vi "AlliGator Compute Average Plot Phasor.vi"(8 "error in (no error)":errorcluster, 9 "Phasor Frequency":dbl[unit]=160000000.0 format="%#_4g", 10 "Mouse Click Coordinates":T2, 11 "XYGraph Ref":refnum<vi>) -> (0 "error out":errorcluster, 1 "Result String":string, 2 "Phasor SDV (g, s)":T1, 3 "Phasor (g, s)":T1)   [LabVIEW 2021, in "AlliGator Phasor Graph.lvlib"]
doc: "Computes average phasor of a single, selected or all phasor plots in the Phasor Graph."
uses:
  AlliGator Phasor Graph.lvlib
  <vilib>/Utility/miscctls.llb/LVPoint32TypeDef.ctl
  Phasor/Phasor (g, s).ctl
  Graphs/Get Plot at Mouse Click (XY Graph)/Get Plot at Mouse Click [AAC].vi
  <userlib>/_OpenG.lib/array/array.llb/Filter 1D Array with Scalar (I32)__ogtk.vi
  <userlib>/_OpenG.lib/array/array.llb/Filter 1D Array (DBL)__ogtk.vi
  Graphs/Graphs.lvlib
  Phasor/Phasor.lvlib
  <vilib>/Analysis/NI_AALBase.lvlib
  Arrays/Arrays.lvlib
  Strings/Strings.lvlib
  Graphs/XY Graph/XY Graph Add-Ons.lvlib
  Phasor Ratio/AlliGator Phasor Ratio.lvlib
  <userlib>/_OpenG.lib/array/array.llb/openg_array.lvlib
  Utilities/Utilities.lvlib
panel:
  # "see the AlliGator License on the block diagram (Ctrl+E or Window:Show Block Diagram)"
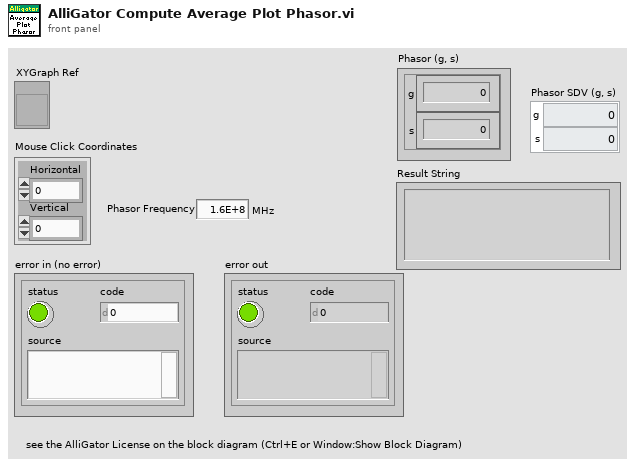
[diagram p1: front panel]
types:
  T1 = typedef "Phasor.lvlib/Phasor (g, s).ctl" = cluster{"g":dbl, "s":dbl}
  T2 = typedef "LVPoint32TypeDef.ctl" = cluster{"Horizontal":i32, "Vertical":i32}
  T3 = typedef "XY Graph Add-Ons.lvlib/XY Graph Refnum.ctl" = refnum<vi>
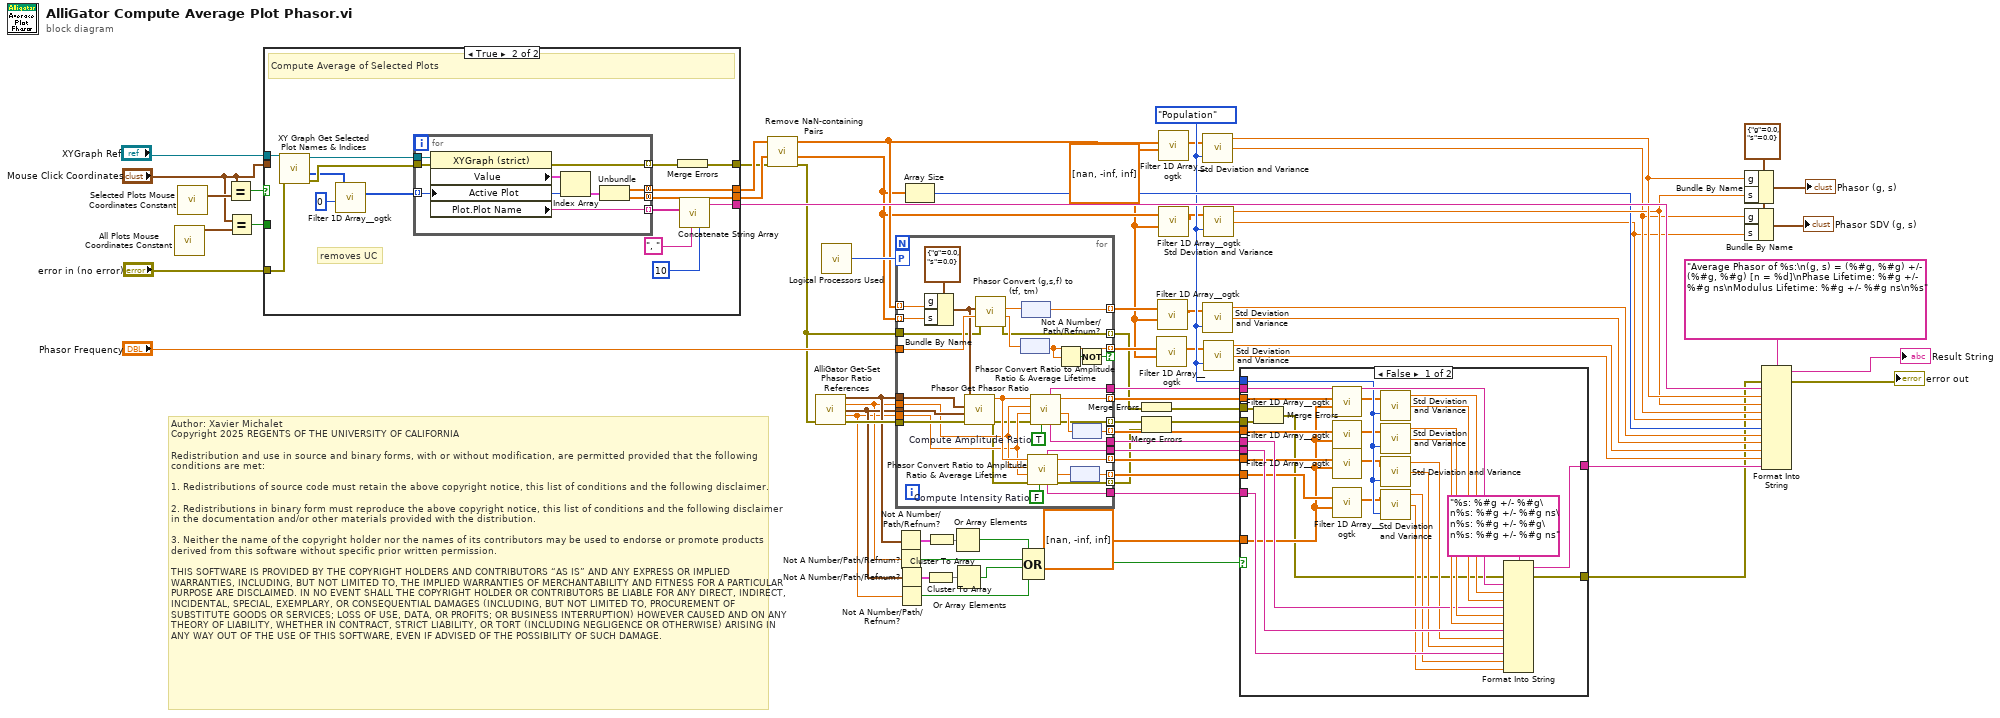
[diagram p0: block diagram]
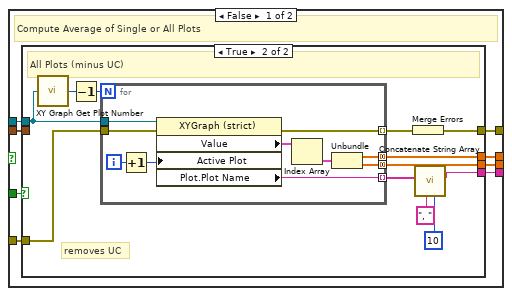
[diagram p3: hidden frame]
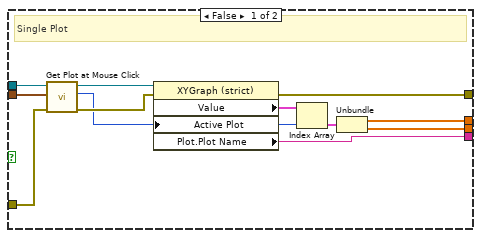
[diagram p4: hidden frame]
diagram:
  w9 = dbl[] [nan, -inf, inf] ("Element(s) to Remove")
  w29 = enum16{"Sample", "Population"}."Population" ("Weighting (Sample)")
  w50 = T1 {"g"=0.0, "s"=0.0} ("Phasor (g, s)")
  # "Author: Xavier Michalet\nCopyright 2025 REGENTS OF THE UNIVERSITY OF CALIFORNIA\n\nRedistribution and use in source and binary forms, with or without modification, are permitted provided that the following conditions are met:\n\n1. Redistributions of source code must retain the above copyright notice, this list of conditions and the following disclaimer.\n\n2. Redistributions in binary form must reproduce the above copyright notice, this list of conditions and the following disclaimer in the documentation and/or other materials provided with the distribution.\n\n3. Neither the name of the copyright holder nor the names of its contributors may be used to endorse or promote products derived from this software without specific prior written permission.\n\nTHIS SOFTWARE IS PROVIDED BY THE COPYRIGHT HOLDERS AND CONTRIBUTORS “AS IS” AND ANY EXPRESS OR IMPLIED WARRANTIES, INCLUDING, BUT NOT LIMITED TO, THE IMPLIED WARRANTIES OF MERCHANTABILITY AND FITNESS FOR A PARTICULAR PURPOSE ARE DISCLAIMED. IN NO EVENT SHALL THE COPYRIGHT HOLDER OR CONTRIBUTORS BE LIABLE FOR ANY DIRECT, INDIRECT, INCIDENTAL, SPECIAL, EXEMPLARY, OR CONSEQUENTIAL DAMAGES (INCLUDING, BUT NOT LIMITED TO, PROCUREMENT OF SUBSTITUTE GOODS OR SERVICES; LOSS OF USE, DATA, OR PROFITS; OR BUSINESS INTERRUPTION) HOWEVER CAUSED AND ON ANY THEORY OF LIABILITY, WHETHER IN CONTRACT, STRICT LIABILITY, OR TORT (INCLUDING NEGLIGENCE OR OTHERWISE) ARISING IN ANY WAY OUT OF THE USE OF THIS SOFTWARE, EVEN IF ADVISED OF THE POSSIBILITY OF SUCH DAMAGE."
  n1 = call "All Plots Mouse Coordinates Constant.vi"() -> ("Selected Plots Mouse Coordinates Equivalent"=w2:T2)
  n2 = call "Selected Plots Mouse Coordinates Constant.vi"() -> ("Selected Plots Mouse Coordinates Equivalent"=w54:T2)
  n3 = Equal?(x="Mouse Click Coordinates", y=w54) -> (x = y?=w53:bool)
  n4 = Equal?(x="Mouse Click Coordinates", y=w2) -> (x = y?=w1:bool)
  n5 = case shown="True" w53 {
    tunnel: "XYGraph Ref" -> [w77 w119]
    tunnel: "error in (no error)" -> [w76 w116]
    tunnel: [w75 w121] -> w66
    tunnel: [w74 w126] -> w62
    tunnel: [w73 w125] -> w61
    tunnel: [w72 w123] -> w60
    tunnel: "Mouse Click Coordinates" -> [w71 _]
    tunnel: w1 -> [w70 _]
    frame False {
      # "Compute Average of Single or All Plots"
      n6 = case shown="True" w70 {
        tunnel: w77 -> [w89 w93]
        tunnel: w76 -> [w88 w92]
        tunnel: [w82 w94] -> w75
        tunnel: [w81 w96] -> w74
        tunnel: [w80 w95] -> w73
        tunnel: [w79 w97] -> w72
        tunnel: w71 -> [w78 _]
        frame False {
          # "Single Plot"
          n7 = call-poly "Get Plot at Mouse Click.vi"("error in (no error)"=w88, "Mouse Click Coordinates"=w78, "XYGraph Ref"=w89) -> ("error out"=w86:errorcluster, "Plot at Coordinates"=w83:i32, "XYGraph Ref"=w87:T3)  [unwired: 2 in, 4 out]
          n8 = property class="XYGraph (strict)"(reference=w87, error in=w86, "Active Plot"=w83) -> (error out=w79:errorcluster, "Value"=w85:cluster{"X Array":dbl[], "Y Array":dbl[]}[], "Plot.Plot Name"=w82:string)  [unwired: 1 out]
          n9 = Index Array(array=w85, index=w83) -> (element=w84:cluster{"X Array":dbl[], "Y Array":dbl[]})
          n10 = Unbundle(w84) -> ("X Array"=w81:dbl[], "Y Array"=w80:dbl[])
        }
        frame True {
          # "removes UC"
          # "All Plots (minus UC)"
          n11 = call "XY Graph Get Plot Number.vi"("XYGraph"=w93) -> ("# Plots"=w91:i32)  [unwired: 8 in]
          n12 = Decrement(x=w91) -> (x-1=w90:i32)
          n13 = for {
            N: w90 -> [_]
            tunnel: [w109] -> w100 mode=indexing
            tunnel: [w108] -> w96 mode=concatenating
            tunnel: [w107] -> w95 mode=concatenating
            tunnel: [w106] -> w101 mode=indexing
            tunnel: w93 -> [w105]
            tunnel: w92 -> [w104]
            i -> [w103]
            n14 = Increment(x=w103) -> (x+1=w102:i32)
            n15 = property class="XYGraph (strict)"(reference=w105, error in=w104, "Active Plot"=w102) -> (error out=w106:errorcluster, "Value"=w111:cluster{"X Array":dbl[], "Y Array":dbl[]}[], "Plot.Plot Name"=w109:string)  [unwired: 1 out]
            n16 = Index Array(array=w111) -> (element=w110:cluster{"X Array":dbl[], "Y Array":dbl[]})  [unwired: 1 in]
            n17 = Unbundle(w110) -> ("X Array"=w108:dbl[], "Y Array"=w107:dbl[])
          }
          n18 = Merge Errors(w101) -> (w97:errorcluster)
          n19 = call "Concatenate String Array.vi"("Max Number of Elements (None: -1)"=10, "Separator (TAB)"=", ", "String Array"=w100) -> ("Formatted String"=w94:string)  [unwired: 8 in]
        }
      }
    }
    frame True {
      # "removes UC"
      # "Compute Average of Selected Plots"
      n20 = call "XY Graph Get Selected Plot Names & Indices.vi"("error in (no error)"=w116, "XYGraph in"=w119) -> ("error out"=w117:errorcluster, "Selected Plots"=w115:i32[], "XYGraph out"=w118:T3)  [unwired: 5 in, 2 out]
      n21 = call-poly <userlib>:"Filter 1D Array__ogtk.vi"("items to filter"=0, "array"=w115) -> ("filtered array"=w113:i32[])  [unwired: 4 in, 1 out]
      n22 = for {
        tunnel: [w133] -> w122 mode=indexing
        tunnel: [w132] -> w126 mode=concatenating
        tunnel: [w131] -> w125 mode=concatenating
        tunnel: [w130] -> w124 mode=indexing
        tunnel: w118 -> [w129]
        tunnel: w117 -> [w128]
        tunnel: w113 -> [w127] mode=indexing
        n23 = property class="XYGraph (strict)"(reference=w129, error in=w128, "Active Plot"=w127) -> (error out=w130:errorcluster, "Value"=w135:cluster{"X Array":dbl[], "Y Array":dbl[]}[], "Plot.Plot Name"=w133:string)  [unwired: 1 out]
        n24 = Index Array(array=w135, index=w127) -> (element=w134:cluster{"X Array":dbl[], "Y Array":dbl[]})
        n25 = Unbundle(w134) -> ("X Array"=w132:dbl[], "Y Array"=w131:dbl[])
      }
      n26 = Merge Errors(w124) -> (w123:errorcluster)
      n27 = call "Concatenate String Array.vi"("Max Number of Elements (None: -1)"=10, "Separator (TAB)"=", ", "String Array"=w122) -> ("Formatted String"=w121:string)  [unwired: 8 in]
    }
  }
  n28 = call "Remove NaN-containing Pairs.vi"("Error In"=w60, "Y Array in"=w61, "X Array in"=w62) -> ("Error Out"=w6:errorcluster, "Y Array out"=w15:dbl[], "X Array out"=w17:dbl[])  [unwired: 5 in, 1 out]
  n29 = call "AlliGator Get-Set Phasor Ratio References.vi"("error in (no error)"=w6) -> ("Reference Phasor 1"=w43:T1, "Reference Lifetime 1"=w40:dbl[unit], "Reference Phasor 2"=w41:T1, "Reference Lifetime 2"=w39:dbl[unit], "error out"=w47:errorcluster)  [unwired: 7 in, 3 out]
  n30 = call "Logical Processors Used.vi"() -> ("# Logical Processor Used"=w23:i32)  [unwired: 6 in]
  n31 = for {
    tunnel: w15 -> [w167] mode=indexing
    tunnel: w17 -> [w168] mode=indexing
    tunnel: "Phasor Frequency" -> [w165]
    tunnel: [w166] -> w13 mode=indexing
    tunnel: [w162] -> w11 mode=indexing if=w160
    tunnel: w47 -> [w159]
    tunnel: w41 -> [w158]
    tunnel: w43 -> [w157]
    tunnel: w39 -> [w146]
    tunnel: w40 -> [w147]
    tunnel: [w155] -> w30 mode=indexing
    tunnel: [w154] -> w45
    tunnel: [w150] -> w46 mode=indexing
    tunnel: [w152] -> w28 mode=indexing
    tunnel: [w151] -> w26
    workers-P: w23 -> [_]
    tunnel: [w143] -> w22
    tunnel: [w142] -> w21 mode=indexing
    tunnel: [w140] -> w20 mode=indexing
    tunnel: [w139] -> w7 mode=indexing
    tunnel: [w138] -> w19
    tunnel: w6 -> [w137]
    tunnel: [w136] -> w5 mode=indexing
    w144 = FALSE  # Compute Intensity Ratio
    w149 = TRUE  # Compute Amplitude Ratio
    n32 = Bundle By Name(cluster=T1 {"g"=0.0, "s"=0.0} ("Phasor (g, s)"), "g"=w168, "s"=w167) -> (w156:T1)
    n33 = call "Phasor Get Phasor Ratio.vi"("Error In"=w159, "Reference Phasor 2"=w158, "Reference Phasor 1"=w157, "Phasor"=w156) -> ("Error Out"=w145:errorcluster, "Phasor Ratio (f1)"=w148:dbl)  [unwired: 5 in, 1 out]
    n34 = call "Phasor Convert (g,s,f) to (tf, tm).vi"("Error In"=w137, "Phasor Harmonic Frequency"=w165, "Phasor (g, s)"=w156) -> ("Error Out"=w136:errorcluster, "Modulus Lifetime"=w163:dbl[unit], "Phase Lifetime"=w164:dbl[unit])  [unwired: 6 in]
    n35 = node(w163) -> (w162:dbl)
    n36 = node(w164) -> (w166:dbl)
    n37 = call "Phasor Convert Ratio to Amplitude Ratio & Average Lifetime.vi"("Compute Amplitude Ratio"=w144, "error in (no error)"=w145, "Reference Lifetime 2"=w146, "Reference Lifetime 1"=w147, "Phasor Ratio (f1)"=w148) -> ("error out"=w139:errorcluster, "Average Lifetime"=w141:dbl[unit], "Phasor/Amplitude Ratio"=w142:dbl, "Average Lifetime Caption"=w138:string, "Phasor Ratio Plot Name Suffix"=w143:string)  [unwired: 2 in]
    n38 = call "Phasor Convert Ratio to Amplitude Ratio & Average Lifetime.vi"("Compute Amplitude Ratio"=w149, "error in (no error)"=w145, "Reference Lifetime 2"=w146, "Reference Lifetime 1"=w147, "Phasor Ratio (f1)"=w148) -> ("error out"=w152:errorcluster, "Average Lifetime"=w153:dbl[unit], "Phasor/Amplitude Ratio"=w155:dbl, "Average Lifetime Caption"=w151:string, "Phasor Ratio Plot Name Suffix"=w154:string)  [unwired: 2 in]
    n39 = Not A Number/Path/Refnum?(number/path/refnum=w162) -> (NaN/Path/Refnum?=w161:bool)
    n40 = node(w141) -> (w140:dbl)
    n41 = node(w153) -> (w150:dbl)
    n42 = Not(x=w161) -> (.not. x?=w160:bool)
  }
  n43 = Not A Number/Path/Refnum?(number/path/refnum=w43) -> (NaN/Path/Refnum?=w42:cluster{"g":bool, "s":bool})
  n44 = Not A Number/Path/Refnum?(number/path/refnum=w40) -> (NaN/Path/Refnum?=w36:bool)
  n45 = Not A Number/Path/Refnum?(number/path/refnum=w41) -> (NaN/Path/Refnum?=w38:cluster{"g":bool, "s":bool})
  n46 = Not A Number/Path/Refnum?(number/path/refnum=w39) -> (NaN/Path/Refnum?=w34:bool)
  n47 = Array Size(array=w15) -> (size(s)=w63:i32)
  n48 = Cluster To Array(cluster=w38) -> (array=w35:bool[])
  n49 = Cluster To Array(cluster=w42) -> (array=w37:bool[])
  n50 = Or Array Elements(Boolean array=w37) -> (logical OR=w33:bool)
  n51 = Or Array Elements(Boolean array=w35) -> (logical OR=w32:bool)
  n52 = Compound Arithmetic op=OR(w33, w36, w32, w34) -> (w31:bool)
  n53 = Merge Errors(w5) -> (w4:errorcluster)
  n54 = Merge Errors(w28, w7) -> (w8:errorcluster)
  n55 = call-poly <userlib>:"Filter 1D Array__ogtk.vi"("items to filter"=w9, "array"=w11) -> ("filtered array"=w10:dbl[])  [unwired: 4 in, 1 out]
  n56 = call-poly <userlib>:"Filter 1D Array__ogtk.vi"("items to filter"=w9, "array"=w13) -> ("filtered array"=w12:dbl[])  [unwired: 4 in, 1 out]
  n57 = call-poly <userlib>:"Filter 1D Array__ogtk.vi"("items to filter"=w9, "array"=w17) -> ("filtered array"=w16:dbl[])  [unwired: 4 in, 1 out]
  n58 = call-poly <userlib>:"Filter 1D Array__ogtk.vi"("items to filter"=w9, "array"=w15) -> ("filtered array"=w14:dbl[])  [unwired: 4 in, 1 out]
  n59 = call <vilib>:"Std Deviation and Variance.vi"("X"=w16, "Weighting (Sample)"=w29) -> ("mean"=w65:dbl, "standard deviation"=w52:dbl)  [unwired: 1 out]
  n60 = call <vilib>:"Std Deviation and Variance.vi"("X"=w12, "Weighting (Sample)"=w29) -> ("mean"=w58:dbl, "standard deviation"=w57:dbl)  [unwired: 1 out]
  n61 = call <vilib>:"Std Deviation and Variance.vi"("X"=w14, "Weighting (Sample)"=w29) -> ("mean"=w64:dbl, "standard deviation"=w51:dbl)  [unwired: 1 out]
  n62 = call <vilib>:"Std Deviation and Variance.vi"("X"=w10, "Weighting (Sample)"=w29) -> ("mean"=w56:dbl, "standard deviation"=w55:dbl)  [unwired: 1 out]
  n63 = case shown="False" w31 {
    tunnel: w46 -> [w178 _]
    tunnel: w45 -> [w196 _]
    tunnel: [w193 _] -> w44
    tunnel: w30 -> [w180 _]
    tunnel: w29 -> [w187 _]
    tunnel: w8 -> [w190 _]
    tunnel: [w189 w198] -> w27
    tunnel: w26 -> [w188 _]
    tunnel: w22 -> [w186 _]
    tunnel: w21 -> [w176 _]
    tunnel: w20 -> [w174 _]
    tunnel: w19 -> [w185 _]
    tunnel: dbl[] [nan, -inf, inf] ("Element(s) to Remove") -> [w172 _]
    tunnel: w4 -> [w170 w198]
    frame False {
      n64 = Merge Errors(w170, w190) -> (w171:errorcluster)
      n65 = call-poly <userlib>:"Filter 1D Array__ogtk.vi"("items to filter"=w172, "array"=w180) -> ("filtered array"=w179:dbl[])  [unwired: 4 in, 1 out]
      n66 = call-poly <userlib>:"Filter 1D Array__ogtk.vi"("items to filter"=w172, "array"=w178) -> ("filtered array"=w177:dbl[])  [unwired: 4 in, 1 out]
      n67 = call-poly <userlib>:"Filter 1D Array__ogtk.vi"("items to filter"=w172, "array"=w176) -> ("filtered array"=w175:dbl[])  [unwired: 4 in, 1 out]
      n68 = call-poly <userlib>:"Filter 1D Array__ogtk.vi"("items to filter"=w172, "array"=w174) -> ("filtered array"=w173:dbl[])  [unwired: 4 in, 1 out]
      n69 = call <vilib>:"Std Deviation and Variance.vi"("X"=w179, "Weighting (Sample)"=w187) -> ("mean"=w192:dbl, "standard deviation"=w191:dbl)  [unwired: 1 out]
      n70 = call <vilib>:"Std Deviation and Variance.vi"("X"=w177, "Weighting (Sample)"=w187) -> ("mean"=w195:dbl, "standard deviation"=w194:dbl)  [unwired: 1 out]
      n71 = call <vilib>:"Std Deviation and Variance.vi"("X"=w175, "Weighting (Sample)"=w187) -> ("mean"=w184:dbl, "standard deviation"=w183:dbl)  [unwired: 1 out]
      n72 = call <vilib>:"Std Deviation and Variance.vi"("X"=w173, "Weighting (Sample)"=w187) -> ("mean"=w182:dbl, "standard deviation"=w181:dbl)  [unwired: 1 out]
      n73 = Format Into String(format string="%s: %#g +/- %#g\n%s: %#g +/- %#g ns\n%s: %#g +/- %#g\n%s: %#g +/- %#g ns", error in=w171, w196, w192, w191, w188, w195, w194, w186, w184, w183, w185, w182, w181) -> (resulting string=w193:string, error out=w189:errorcluster)  [unwired: 1 in]
    }
    frame True {
    }
  }
  n74 = Bundle By Name(cluster=w50, "g"=w65, "s"=w64) -> (→"Phasor (g, s)":T1)
  n75 = Bundle By Name(cluster=w50, "g"=w52, "s"=w51) -> (→"Phasor SDV (g, s)":T1)
  n76 = Format Into String(format string="Average Phasor of %s:\n(g, s) = (%#g, %#g) +/- (%#g, %#g) [n = %d]\nPhase Lifetime: %#g +/- %#g ns\nModulus Lifetime: %#g +/- %#g ns\n%s" ("initial string"), error in=w27, w66, w65, w64, w52, w51, w63, w58, w57, w56, w55, w44) -> (resulting string=→"Result String":string, error out=→"error out":errorcluster)  [unwired: 1 in]
